vi "solar Menu TargetsLB.vi"(6 "MenuRef (Activation only)":refnum<k9>, 7 "SOLAR Refnum":T1, 8 "error in (no error)":errorcluster, 9 "ItemTag (Selection only)":string, 10 "Coords":T2, 11 "ListBox in":refnum<vi>) -> (0 "error out":errorcluster)   [LabVIEW 2018]
doc: "This initializes the right-click menu for the Targets listbox."
uses:
  <vilib>/Utility/miscctls.llb/LVPoint32TypeDef.ctl
  solar_ctl SOLAR Refnum.ctl
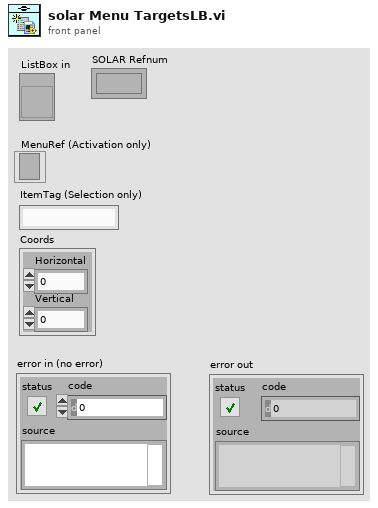
[diagram p1: front panel]
types:
  T1 = typedef "solar_ctl SOLAR Refnum.ctl" = refnum<k1>
  T2 = typedef "LVPoint32TypeDef.ctl" = cluster{"Horizontal":i32, "Vertical":i32}
  T3 = typedef "solar_ctl SOLAR Global.ctl" = cluster{"Targets":T4[], "AppDir":path, "solar.ini":path, "ConfigsDir":path, "CosmosDir":path, "LogsDir":path, "ExePath":path, "ExeVersion":string, "PartNum":string, "AppSetup":string, "Title":string, "Main.ini":path, "Temp.ini":path, "vSOLAR":string, "Splash.png":string, "SplashWait":i32, "SOLARUE":refnum<user-event>, "VoyagerRefnum":T5, "QTimerRefnum":T6}
  T4 = typedef "solar_ctl Target Global.ctl" = cluster{"Target":string, "Q":refnum<queue>, "UE":refnum<user-event>, "VI":refnum<vi>, "Menu":refnum<k9>, "Data":refnum<data-value>, "Attributes":variant}
  T5 = typedef "solar_voy_ctl Voyager Refnum.ctl" = refnum<k1>
  T6 = typedef "solar_qtimer_ctl Refnum.ctl" = refnum<k1>
  T7 = typedef "solar_voy_ctl Voyager.ctl" = cluster{"PACKETS":T8[], "COSMOS_Root":path, "CMD_HDR":T13, "TLM_HDR":T13, "TCPs":T14[], "VoyagerIDOffset":cluster{"VoyagerIDOffset":u16[], "Target Names":string[]}}
  T8 = typedef "solar_voy_def_ctl PACKET.ctl" = cluster{"PACKET_ID":T9, "ENDIAN":enum8{"BIG", "LITTLE"}, "DESC":string, "HZRD":bool, "ITEMS":T10[], "NoExport":bool, "last_time":timestamp, "last_count":u32, "last_data":string}
  T9 = typedef "solar_voy_def_ctl PACKET_ID.ctl" = cluster{"ID":u16, "CMD":enum8{"CMD", "TLM"}, "TARGET":string, "PACKET":string}
  T10 = typedef "solar_voy_def_ctl ITEM.ctl" = cluster{"NAME":string, "OFFSET":i32, "SIZE":i32, "TYPE":T11, "EACH_SIZE":i32, "LVTYPE":T12, "MIN":dbl, "MAX":dbl, "DEFAULT":string, "DESC":string, "ID":bool, "MODIFIERS":variant, "last_value":variant}
  T11 = typedef "solar_voy_def_ctl ITEM TYPE.ctl" = enum8{"BLOCK", "INT", "UINT", "FLOAT", "STRING"}
  T12 = typedef "solar_type Item Type.ctl" = enum16{"NULL", "UNKNOWN", "CLUSTER", "I8", "I16", "I32", "I64", "U8", "U16", "U32", "U64", "U8_ENUM", "U16_ENUM", "U32_ENUM", "SGL", "DBL", "BOOLEAN", "STRING", "PATH", "VISA", "TAG", "TIME", "I8_1D", "I16_1D", "I32_1D", "I64_1D", "U8_1D", "U16_1D", "U32_1D", "U64_1D", "U8_ENUM_1D", "U16_ENUM_1D", "U32_ENUM_1D", "SGL_1D", "DBL_1D", "BOOLEAN_1D", "STRING_1D", "PATH_1D", "VISA_1D", "TAG_1D", "TIME_1D", "I8_2D", "I16_2D", "I32_2D", "I64_2D", "U8_2D", "U16_2D", "U32_2D", "U64_2D", "U8_ENUM_2D", "U16_ENUM_2D", "U32_ENUM_2D", "SGL_2D", "DBL_2D", "BOOLEAN_2D", "STRING_2D", "PATH_2D", "VISA_2D", "TAG_2D", "TIME_2D"}
  T13 = typedef "solar_voy_def_ctl HDR.ctl" = cluster{"ITEMS":T10[], "LENGTH_NAME":string, "LENGTH_VALUE_OFFSET":i32, "ID_NAME":string, "ENDIAN":enum8{"BIG", "LITTLE"}, "GUID_NAME":string, "DEFAULT_TARGET":string, "DEFAULT_PACKET":string, "DEFAULT_ERROR":string}
  T14 = typedef "solar_voy_ctl TCP.ctl" = cluster{"Connected":bool, "Port":u16, "Listener":refnum<k5>, "ServerIP":string, "TCP":refnum<k5>, "Setup":T15, "VIRefnum":refnum<vi>, "TARGETS_CMD":string[], "TARGETS_TLM":string[]}
  T15 = typedef "solar_voy_ctl Port Setup.ctl" = enum8{"SERVER", "CLIENT", "SERVER_CMD", "SERVER_TLM"}
  T16 = typedef "solar_qtimer_ctl QTimer.ctl" = cluster{"Settings":T17, "Queue":refnum<queue>, "QTimerQ":refnum<queue>, "VI Refnum":refnum<vi>}
  T17 = typedef "solar_qtimer_ctl QTimer Settings.ctl" = cluster{"QTimer":string, "Delay":i32, "Start":bool, "EnQ_Type":enum8{"Normal", "Priority", "IgnoreIfExists"}, "Messages":cluster{"MSG":string, "DATA":variant}[]}
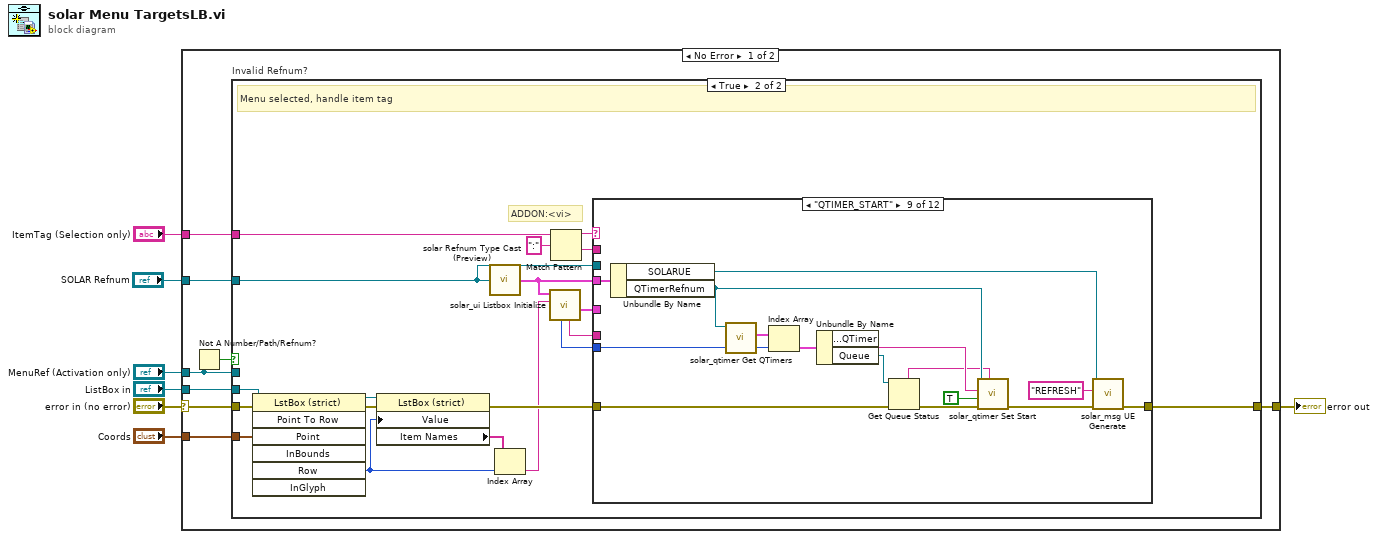
[diagram p0: block diagram]
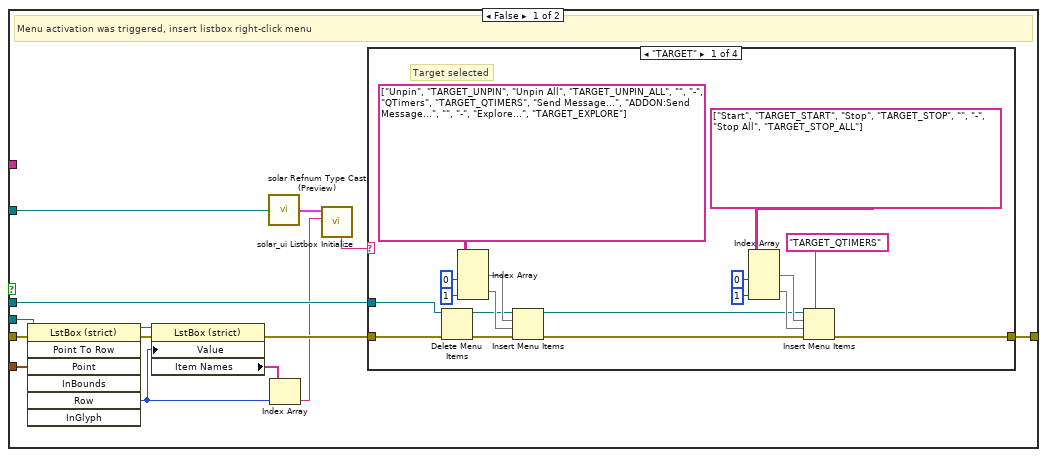
[diagram p2: hidden frame]
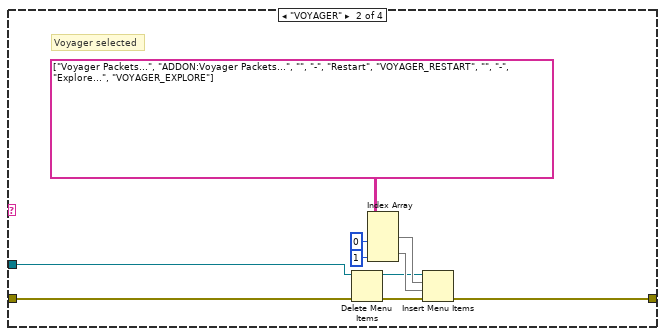
[diagram p3: hidden frame]
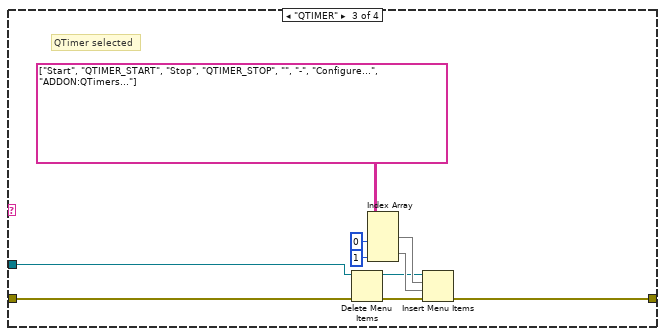
[diagram p4: hidden frame]
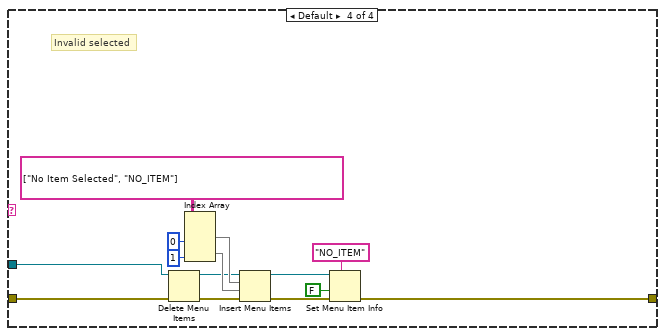
[diagram p5: hidden frame]
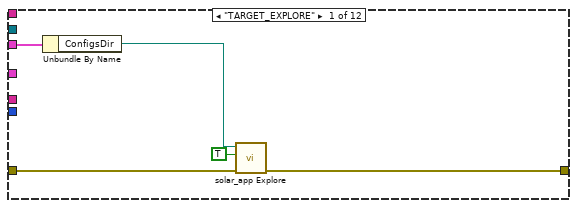
[diagram p6: hidden frame]
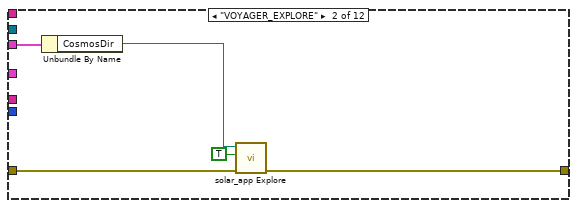
[diagram p7: hidden frame]
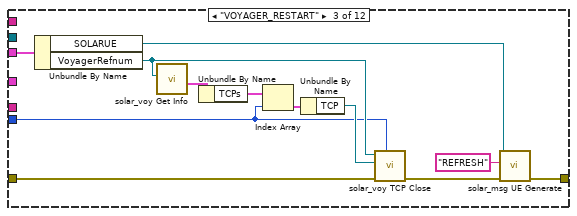
[diagram p8: hidden frame]
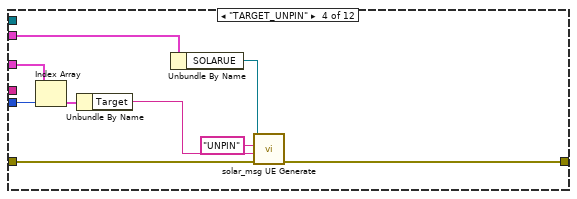
[diagram p9: hidden frame]
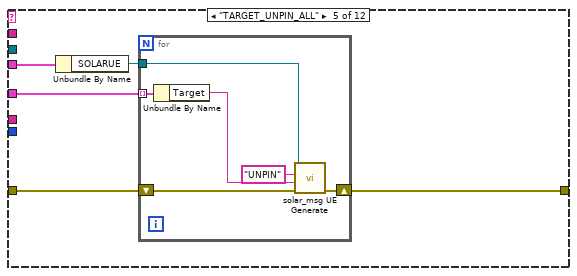
[diagram p10: hidden frame]
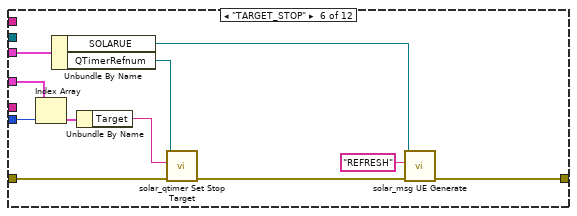
[diagram p11: hidden frame]
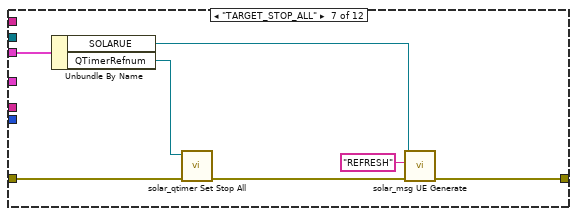
[diagram p12: hidden frame]
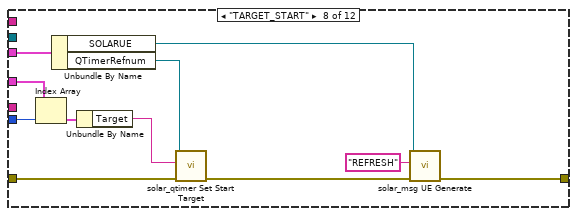
[diagram p13: hidden frame]
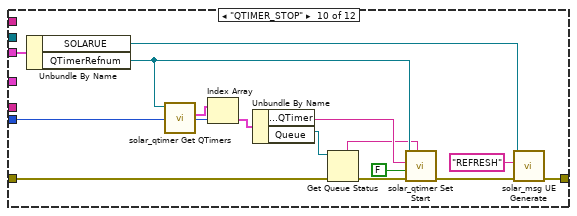
[diagram p14: hidden frame]
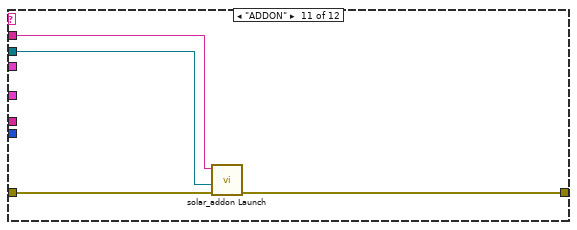
[diagram p15: hidden frame]
diagram:
  n1 = case shown="No Error" "error in (no error)" {
    selector: "error in (no error)" -> [w13 w207]
    tunnel: "Coords" -> [w15 _]
    tunnel: "ListBox in" -> [w14 _]
    tunnel: [w12 w207] -> w4
    tunnel: "MenuRef (Activation only)" -> [w11 _]
    tunnel: "ItemTag (Selection only)" -> [w9 _]
    tunnel: "SOLAR Refnum" -> [w8 _]
    frame No Error {
      n2 = Not A Number/Path/Refnum?(number/path/refnum=w11) -> (NaN/Path/Refnum?=w10:bool)
      n3 = case "Invalid Refnum?" shown="True" w10 {
        tunnel: w15 -> [w26 w95]
        tunnel: w14 -> [w25 w94]
        tunnel: w11 -> [w24 _]
        tunnel: w13 -> [w23 w97]
        tunnel: [w22 w100] -> w12
        tunnel: w9 -> [_ w86]
        tunnel: w8 -> [w18 w82]
        frame False {
          # "Menu activation was triggered, insert listbox right-click menu"
          n4 = invoke class="LstBox (strict)" method="Point To Row"(reference=w25, error in=w23, "Point"=w26) -> (reference out=w27:refnum<vi>, error out=w28:errorcluster, "Row"=w20:i32)  [unwired: 4 in, 4 out]
          n5 = property class="LstBox (strict)"(reference=w27, error in=w28, "Value"=w20) -> (error out=w29:errorcluster, "Item Names"=w21:string[])  [unwired: 1 out]
          n6 = call "solar Refnum Type Cast (Preview).vi"("Refnum"=w18) -> ("SOLAR"=w17:T3)  [unwired: 8 in]
          n7 = Index Array(array=w21, index=w20) -> (element=w19:string)
          n8 = call "solar_ui Listbox Initialize.vi"("Selected Listbox Item"=w19, "SOLAR"=w17) -> ("Selected Item Type"=w16:string)  [unwired: 4 in, 5 out]
          n9 = case shown="\"TARGET\"" w16 {
            tunnel: w29 -> [w47 w57 w67 w81]
            tunnel: w24 -> [w39 w49 w59 w73]
            tunnel: [w31 w48 w58 w71] -> w22
            frame "TARGET" {
              # "Target selected"
              n10 = Delete Menu Items(6:w47, 9:w39) -> (0:w41:errorcluster, 3:w40:refnum<k9>)  [unwired: 2 in]
              n11 = Index Array(array=string[][] [["Unpin", "TARGET_UNPIN"], ["Unpin All", "TARGET_UNPIN_ALL"], ["", "-"], ["QTimers", "TARGET_QTIMERS"], ["Send Message...", "ADDON:Send Message..."], ["", "-"], ["Explore...", "TARGET_EXPLORE"]], index (col) #1=0 ("disabled index (col)"), index (col) #2=1 ("index (col)")) -> (element #1=w45:string[], element #2=w46:string[])  [unwired: 2 in]
              n12 = Insert Menu Items(6:w41, 7:w46, 8:w45, 9:w40) -> (0:w34:errorcluster, 3:w33:refnum<k9>)  [unwired: 2 in, 1 out]
              n13 = Index Array(array=string[][] [["Start", "TARGET_START"], ["Stop", "TARGET_STOP"], ["", "-"], ["Stop All", "TARGET_STOP_ALL"]], index (col) #1=0 ("disabled index (col)"), index (col) #2=1 ("index (col)")) -> (element #1=w36:string[], element #2=w35:string[])  [unwired: 2 in]
              n14 = Insert Menu Items(5:"TARGET_QTIMERS", 6:w34, 7:w35, 8:w36, 9:w33) -> (0:w31:errorcluster)  [unwired: 1 in, 2 out]
            }
            frame "VOYAGER" {
              # "Voyager selected"
              n15 = Delete Menu Items(6:w57, 9:w49) -> (0:w51:errorcluster, 3:w50:refnum<k9>)  [unwired: 2 in]
              n16 = Index Array(array=string[][] [["Voyager Packets...", "ADDON:Voyager Packets..."], ["", "-"], ["Restart", "VOYAGER_RESTART"], ["", "-"], ["Explore...", "VOYAGER_EXPLORE"]], index (col) #1=0 ("disabled index (col)"), index (col) #2=1 ("index (col)")) -> (element #1=w55:string[], element #2=w56:string[])  [unwired: 2 in]
              n17 = Insert Menu Items(6:w51, 7:w56, 8:w55, 9:w50) -> (0:w48:errorcluster)  [unwired: 2 in, 2 out]
            }
            frame "QTIMER" {
              # "QTimer selected"
              n18 = Delete Menu Items(6:w67, 9:w59) -> (0:w61:errorcluster, 3:w60:refnum<k9>)  [unwired: 2 in]
              n19 = Index Array(array=string[][] [["Start", "QTIMER_START"], ["Stop", "QTIMER_STOP"], ["", "-"], ["Configure...", "ADDON:QTimers..."]], index (col) #1=0 ("disabled index (col)"), index (col) #2=1 ("index (col)")) -> (element #1=w65:string[], element #2=w66:string[])  [unwired: 2 in]
              n20 = Insert Menu Items(6:w61, 7:w66, 8:w65, 9:w60) -> (0:w58:errorcluster)  [unwired: 2 in, 2 out]
            }
            frame Default {
              # "Invalid selected"
              n21 = Delete Menu Items(6:w81, 9:w73) -> (0:w75:errorcluster, 3:w74:refnum<k9>)  [unwired: 2 in]
              n22 = Index Array(array=string[][] [["No Item Selected", "NO_ITEM"]], index (col) #1=0 ("disabled index (col)"), index (col) #2=1 ("index (col)")) -> (element #1=w79:string[], element #2=w80:string[])  [unwired: 2 in]
              n23 = Insert Menu Items(6:w75, 7:w80, 8:w79, 9:w74) -> (0:w72:errorcluster, 3:w70:refnum<k9>)  [unwired: 2 in, 1 out]
              n24 = Set Menu Item Info(7:"NO_ITEM" ("item tag"), 8:w72, 9:FALSE ("enabled"), 11:w70) -> (0:w71:errorcluster)  [unwired: 3 in, 1 out]
            }
          }
        }
        frame True {
          # "ADDON:<vi>"
          # "Menu selected, handle item tag"
          n25 = invoke class="LstBox (strict)" method="Point To Row"(reference=w94, error in=w97, "Point"=w95) -> (reference out=w98:refnum<vi>, error out=w99:errorcluster, "Row"=w92:i32)  [unwired: 4 in, 4 out]
          n26 = property class="LstBox (strict)"(reference=w98, error in=w99, "Value"=w92) -> (error out=w96:errorcluster, "Item Names"=w93:string[])  [unwired: 1 out]
          n27 = call "solar Refnum Type Cast (Preview).vi"("Refnum"=w82) -> ("SOLAR"=w90:T3)  [unwired: 8 in]
          n28 = Index Array(array=w93, index=w92) -> (element=w91:string)
          n29 = call "solar_ui Listbox Initialize.vi"("Selected Listbox Item"=w91, "SOLAR"=w90) -> ("Visible Targets"=w89:T4[], "Selected Item Type"=w88:string, "Relative Index of Item"=w87:i32)  [unwired: 4 in, 3 out]
          n30 = Match Pattern(string=w86, regular expression=":") -> (before substring=w85:string, after substring=w83:string)  [unwired: 1 in, 2 out]
          n31 = case shown="\"QTIMER_START\"" w85 {
            tunnel: w90 -> [w105 w110 w122 w131 w136 w153 w160 w171 w186 w201 _ _]
            tunnel: [w103 w108 w112 w129 w134 w144 w158 w162 w178 w193 w204 w206] -> w100
            tunnel: w96 -> [w104 w109 w119 w130 w135 w149 w156 w167 w184 w199 w205 w206]
            tunnel: w89 -> [_ _ _ w126 w132 w152 _ w170 _ _ _ _]
            tunnel: w88 -> [_ _ _ _ _ _ _ _ _ _ _ _]
            tunnel: w87 -> [_ _ w115 w125 _ w151 _ w169 w185 w200 _ _]
            tunnel: w83 -> [_ _ _ _ _ _ _ _ _ _ w203 _]
            tunnel: w82 -> [_ _ _ _ _ _ _ _ _ _ w202 _]
            frame "TARGET_EXPLORE" {
              n32 = Unbundle By Name(w105) -> ("ConfigsDir"=w102:path)
              n33 = call "solar_app Explore.vi"("error in (no error)"=w104, "Open Folder? (F)"=TRUE, "File or Folder Path"=w102) -> ("error out"=w103:errorcluster)  [unwired: 8 in]
            }
            frame "VOYAGER_EXPLORE" {
              n34 = Unbundle By Name(w110) -> ("CosmosDir"=w107:path)
              n35 = call "solar_app Explore.vi"("error in (no error)"=w109, "Open Folder? (F)"=TRUE, "File or Folder Path"=w107) -> ("error out"=w108:errorcluster)  [unwired: 8 in]
            }
            frame "VOYAGER_RESTART" {
              n36 = Unbundle By Name(w122) -> ("SOLARUE"=w111:refnum<user-event>, "VoyagerRefnum"=w120:T5)
              n37 = call "solar_voy Get Info.vi"("Voyager Refnum"=w120) -> ("Voyager"=w121:T7)  [unwired: 8 in, 2 out]
              n38 = Unbundle By Name(w121) -> ("TCPs"=w118:T14[])
              n39 = Index Array(array=w118, index=w115) -> (element=w117:T14)
              n40 = Unbundle By Name(w117) -> ("TCP"=w116:refnum<k5>)
              n41 = call "solar_voy TCP Close.vi"("Instance"=w115, "error in (no error)"=w119, "Connection ID"=w116, "Voyager Refnum in"=w120) -> ("error out"=w113:errorcluster)  [unwired: 6 in, 1 out]
              n42 = call "solar_msg UE Generate.vi"("error in (no error)"=w113, "CMD (Last)"="REFRESH", "UserEvent in"=w111) -> ("error out"=w112:errorcluster)  [unwired: 7 in, 1 out]
            }
            frame "TARGET_UNPIN" {
              n43 = Index Array(array=w126, index=w125) -> (element=w124:T4)
              n44 = Unbundle By Name(w124) -> ("Target"=w123:string)
              n45 = Unbundle By Name(w131) -> ("SOLARUE"=w128:refnum<user-event>)
              n46 = call "solar_msg UE Generate.vi"("error in (no error)"=w130, "CMD_DATA (Last)"=w123, "CMD (Last)"="UNPIN", "UserEvent in"=w128) -> ("error out"=w129:errorcluster)  [unwired: 6 in, 1 out]
            }
            frame "TARGET_UNPIN_ALL" {
              n47 = Unbundle By Name(w136) -> ("SOLARUE"=w133:refnum<user-event>)
              n48 = for {
                tunnel: w133 -> [w140]
                shift-right: [w141] -> w134
                shift-left: w135 -> [w142]
                tunnel: w132 -> [w138] mode=indexing
                n49 = Unbundle By Name(w138) -> ("Target"=w137:string)
                n50 = call "solar_msg UE Generate.vi"("error in (no error)"=w142, "CMD_DATA (Last)"=w137, "CMD (Last)"="UNPIN", "UserEvent in"=w140) -> ("error out"=w141:errorcluster)  [unwired: 6 in, 1 out]
              }
            }
            frame "TARGET_STOP" {
              n51 = Index Array(array=w152, index=w151) -> (element=w150:T4)
              n52 = Unbundle By Name(w153) -> ("SOLARUE"=w143:refnum<user-event>, "QTimerRefnum"=w148:T6)
              n53 = Unbundle By Name(w150) -> ("Target"=w147:string)
              n54 = call "solar_qtimer Set Stop Target.vi"("error in (no error)"=w149, "Target (Queue Name)"=w147, "QTimer Refnum in"=w148) -> ("error out"=w145:errorcluster)  [unwired: 5 in, 3 out]
              n55 = call "solar_msg UE Generate.vi"("error in (no error)"=w145, "CMD (Last)"="REFRESH", "UserEvent in"=w143) -> ("error out"=w144:errorcluster)  [unwired: 7 in, 1 out]
            }
            frame "TARGET_STOP_ALL" {
              n56 = Unbundle By Name(w160) -> ("SOLARUE"=w157:refnum<user-event>, "QTimerRefnum"=w154:T6)
              n57 = call "solar_qtimer Set Stop All.vi"("error in (no error)"=w156, "QTimer Refnum in"=w154) -> ("error out"=w155:errorcluster)  [unwired: 6 in, 3 out]
              n58 = call "solar_msg UE Generate.vi"("error in (no error)"=w155, "CMD (Last)"="REFRESH", "UserEvent in"=w157) -> ("error out"=w158:errorcluster)  [unwired: 7 in, 1 out]
            }
            frame "TARGET_START" {
              n59 = Index Array(array=w170, index=w169) -> (element=w168:T4)
              n60 = Unbundle By Name(w171) -> ("SOLARUE"=w161:refnum<user-event>, "QTimerRefnum"=w166:T6)
              n61 = Unbundle By Name(w168) -> ("Target"=w165:string)
              n62 = call "solar_qtimer Set Start Target.vi"("error in (no error)"=w167, "Target (Queue Name)"=w165, "QTimer Refnum in"=w166) -> ("error out"=w163:errorcluster)  [unwired: 5 in, 3 out]
              n63 = call "solar_msg UE Generate.vi"("error in (no error)"=w163, "CMD (Last)"="REFRESH", "UserEvent in"=w161) -> ("error out"=w162:errorcluster)  [unwired: 7 in, 1 out]
            }
            frame "QTIMER_START" {
              n64 = Unbundle By Name(w186) -> ("SOLARUE"=w177:refnum<user-event>, "QTimerRefnum"=w183:T6)
              n65 = call "solar_qtimer Get QTimers.vi"("QTimer Refnum"=w183) -> ("QTimers"=w176:T16[])  [unwired: 8 in, 2 out]
              n66 = Index Array(array=w176, index=w185) -> (element=w182:T16)
              n67 = Unbundle By Name(w182) -> ("Settings.QTimer"=w175:string, "Queue"=w173:refnum<queue>)
              n68 = Get Queue Status(queue=w173, error in (no error)=w184) -> (queue name=w172:string, error out=w174:errorcluster)  [unwired: 1 in, 6 out]
              n69 = call "solar_qtimer Set Start.vi"("Target Name"=w172, "error in (no error)"=w174, "Start (F = Stop)"=TRUE, "QTimer Name"=w175, "QTimer Refnum in"=w183) -> ("error out"=w179:errorcluster)  [unwired: 5 in, 1 out]
              n70 = call "solar_msg UE Generate.vi"("error in (no error)"=w179, "CMD (Last)"="REFRESH", "UserEvent in"=w177) -> ("error out"=w178:errorcluster)  [unwired: 7 in, 1 out]
            }
            frame "QTIMER_STOP" {
              n71 = Unbundle By Name(w201) -> ("SOLARUE"=w192:refnum<user-event>, "QTimerRefnum"=w198:T6)
              n72 = call "solar_qtimer Get QTimers.vi"("QTimer Refnum"=w198) -> ("QTimers"=w191:T16[])  [unwired: 8 in, 2 out]
              n73 = Index Array(array=w191, index=w200) -> (element=w197:T16)
              n74 = Unbundle By Name(w197) -> ("Settings.QTimer"=w190:string, "Queue"=w188:refnum<queue>)
              n75 = Get Queue Status(queue=w188, error in (no error)=w199) -> (queue name=w187:string, error out=w189:errorcluster)  [unwired: 1 in, 6 out]
              n76 = call "solar_qtimer Set Start.vi"("Target Name"=w187, "error in (no error)"=w189, "Start (F = Stop)"=FALSE, "QTimer Name"=w190, "QTimer Refnum in"=w198) -> ("error out"=w194:errorcluster)  [unwired: 5 in, 1 out]
              n77 = call "solar_msg UE Generate.vi"("error in (no error)"=w194, "CMD (Last)"="REFRESH", "UserEvent in"=w192) -> ("error out"=w193:errorcluster)  [unwired: 7 in, 1 out]
            }
            frame "ADDON" {
              n78 = call "solar_addon Launch.vi"("error in (no error)"=w205, "SOLAR Refnum"=w202, "Menu Label"=w203) -> ("error out"=w204:errorcluster)  [unwired: 6 in, 2 out]
            }
            frame Default {
            }
          }
        }
      }
    }
    frame Error {
    }
  }
  "error out" <- w4
